vi "GetPicoMsg.vi"(3 "CfgRef":refnum<vi>) -> (0 "Values":dbl[](array[numeric]), 1 "Data":bool, 2 "Msg":string)   [LabVIEW 2025]
uses:
  Globals.vi
  Range.ctl
  Mode.ctl
  Config.ctl
panel:
  # "R1 Only"
  # "Parallel"
  # "Serial"
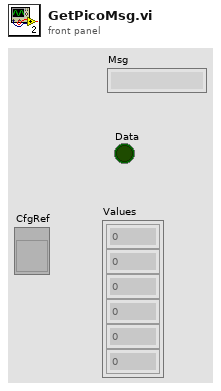
[diagram p1: front panel]
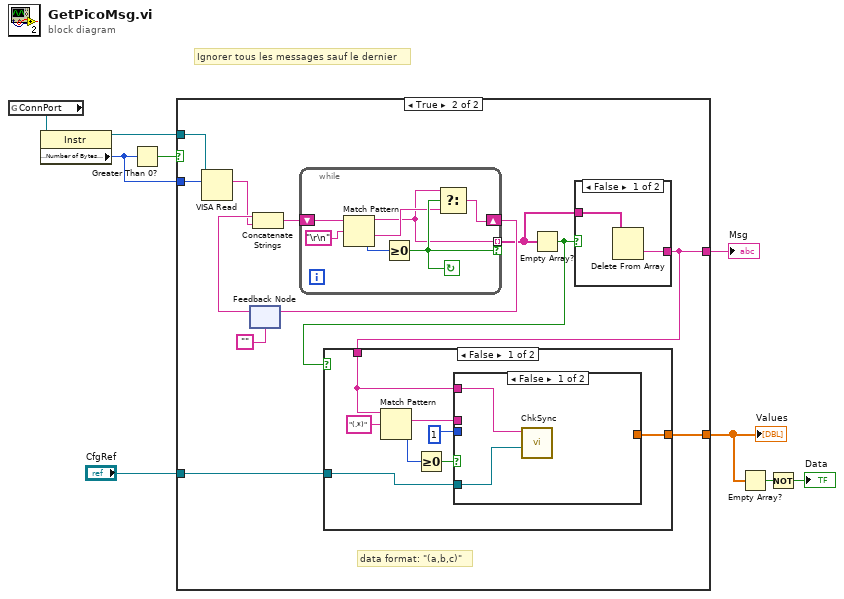
[diagram p0: block diagram]
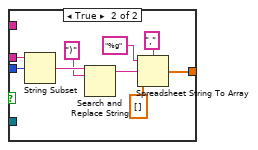
[diagram p3: hidden frame]
diagram:
  # "Ignorer tous les messages sauf le dernier"
  n1 = global read "Globals.vi" "ConnPort"() -> (w9:refnum<visa-resource-name>)
  n2 = property class="Instr"(reference=w9) -> (reference out=w7:refnum<visa-resource-name>, "Serial Settings:Number of Bytes at Serial Port"=w6:u32)  [unwired: 1 in, 1 out]
  n3 = Greater Than 0?(x=w6) -> (x > 0?=w8:bool)
  n4 = case shown="True" w8 {
    tunnel: w7 -> [_ w21]
    tunnel: w6 -> [_ w17]
    tunnel: [_ w12] -> w5
    tunnel: [_ w11] -> w4
    tunnel: "CfgRef" -> [_ w10]
    frame False {
    }
    frame True {
      # "data format: \"(a,b,c)\""
      n5 = VISA Read(VISA resource name=w21, byte count=w17) -> (read buffer=w18:string)  [unwired: 1 in, 3 out]
      n6 = feedback #1("") -> (w19:string)
      n7 = Concatenate Strings(w19, w18) -> (w16:string)
      n8 = while {
        tunnel: [w43] -> w14 mode=indexing if=w45
        shift-right: [w46] -> w15
        shift-left: w16 -> [w48]
        stop <- w45 continue-if-true
        n9 = Match Pattern(string=w48, regular expression="\r\n") -> (before substring=w43:string, after substring=w44:string, offset past match=w47:i32)  [unwired: 1 in, 1 out]
        n10 = Greater Or Equal To 0?(x=w47) -> (x >= 0?=w45:bool)
        n11 = Select(t=w43, s=w45, f=w44) -> (s? t:f=w46:string)
      }
      n12 = feedback-in #1(w15) -> ()
      n13 = Empty Array?(array=w14) -> (empty?=w13:bool)
      n14 = case shown="False" w13 {
        tunnel: w14 -> [w42 _]
        tunnel: [w41 _] -> w12
        frame False {
          n15 = Delete From Array(array=w42) -> (deleted portion=w41:string)  [unwired: 2 in, 1 out]
        }
        frame True {
        }
      }
      n16 = case shown="False" w13 {
        tunnel: w12 -> [w23 _]
        tunnel: [w24 _] -> w11
        tunnel: w10 -> [w22 _]
        frame False {
          n17 = Match Pattern(string=w23, regular expression="(.*)") -> (match substring=w26:string, offset past match=w28:i32)  [unwired: 1 in, 2 out]
          n18 = Greater Or Equal To 0?(x=w28) -> (x >= 0?=w27:bool)
          n19 = case shown="False" w27 {
            tunnel: w26 -> [_ w40]
            tunnel: 1 ("offset (0)") -> [_ w39]
            tunnel: [_ w32] -> w24
            tunnel: w23 -> [w31 _]
            tunnel: w22 -> [w30 _]
            frame False {
              n20 = call "ChkSync.vi"("ConfigReg"=w30, "Msg"=w31) -> ()  [unwired: 10 in]
            }
            frame True {
              n21 = String Subset(string=w40, offset (0)=w39) -> (substring=w38:string)  [unwired: 1 in]
              n22 = Search and Replace String(input string=w38, search string=")") -> (result string=w36:string)  [unwired: 6 in, 3 out]
              n23 = Spreadsheet String To Array(delimiter (Tab)=",", format string="%g" ("delimiter (Tab)"), spreadsheet string=w36, array type (2D Dbl)=dbl[] []) -> (array=w32:dbl[])
            }
          }
        }
        frame True {
        }
      }
    }
  }
  "Msg" <- w5
  "Values" <- w4
  n24 = Empty Array?(array=w4) -> (empty?=w3:bool)
  n25 = Not(x=w3) -> (.not. x?=→"Data":bool)
